vi "Get State.vi"(8 "error in (no error)":errorcluster, 11 "Elevator in":refnum<class "Elevator.lvclass">) -> (0 "error out":errorcluster, 1 "Elevator State String":string, 3 "Elevator out":refnum<class "Elevator.lvclass">)   [LabVIEW 2014, in "Elevator.lvlib" / "Elevator.lvclass"]
uses:
  Elevator.lvclass
  Elevator.lvclass/Elevator.ctl
  Elevator State.ctl
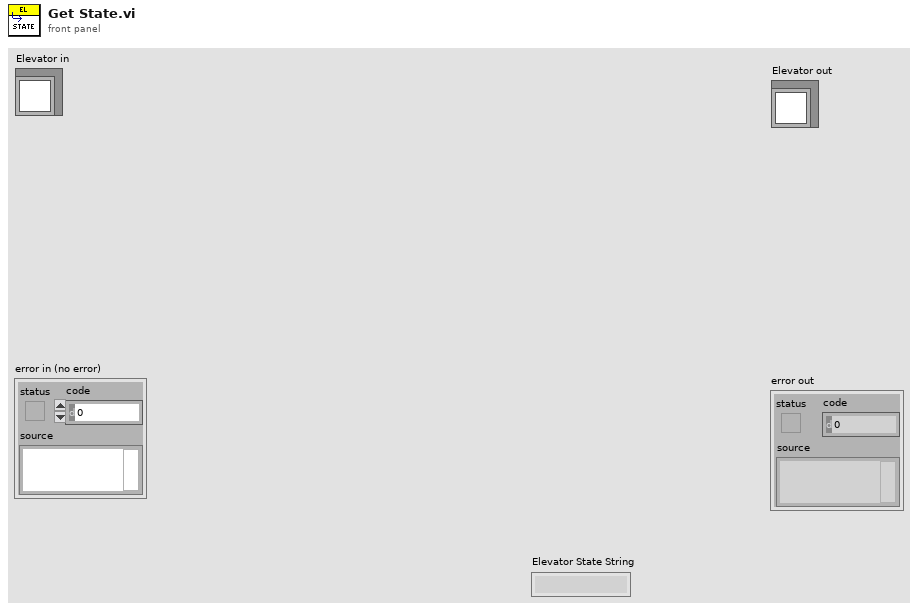
[diagram p1: front panel]
types:
  T1 = typedef "Elevator.lvlib/Elevator.lvclass/Elevator State.ctl" = cluster{"At Bottom":bool, "At Top":bool, "At Setpoint":bool, "Target Rate (RPM)":dbl, "Current Travel Rate":dbl, "Current Elevation":dbl, "Brake On":bool, "Motor Elevate Rate (RPM))":dbl, "Has Been Home":bool}
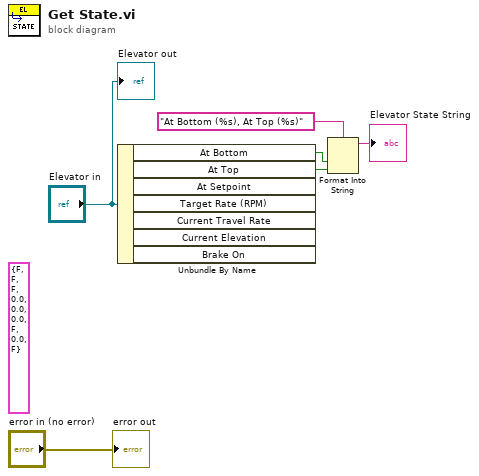
[diagram p0: block diagram]
diagram:
  (unwired) T1 {"At Bottom"=FALSE, "At Top"=FALSE, "At Setpoint"=FALSE, "Target Rate (RPM)"=0.0, "Current Travel Rate"=0.0, "Current Elevation"=0.0, "Brake On"=FALSE, "Motor Elevate Rate (RPM))"=0.0, "Has Been Home"=FALSE} ("Eleveator State")
  n1 = Unbundle By Name("Elevator in") -> ("At Bottom"=w3:bool, "At Top"=w2:bool)  [unwired: 5 out]
  n2 = Format Into String(format string="At Bottom (%s), At Top (%s)", w3, w2) -> (resulting string=→"Elevator State String":string)  [unwired: 2 in, 1 out]
  "error out" <- "error in (no error)"
  "Elevator out" <- "Elevator in"
